vi "user process.vi"(8 "error in":errorcluster, 10 "Parameters to process":T2, 11 "Custom Temperature Controller runtime in":refnum<class "Custom Temperature Controller runtime.lvclass">) -> (0 "error out":errorcluster, 2 "Results from processing":T1, 3 "Custom Temperature Controller runtime out":refnum<class "Custom Temperature Controller runtime.lvclass">)   [LabVIEW 2021, in "Custom Temperature Controller runtime.lvclass"]
uses:
  Custom Temperature Controller runtime.lvclass
  parameter user data.ctl
  result user data.ctl
  Custom Temperature Controller runtime.lvclass/Custom Temperature Controller runtime.ctl
  <vilib>/addons/control/pid/pid.llb/PID (DBL).vi
  <vilib>/addons/control/pid/NI_PID_pid.lvlib
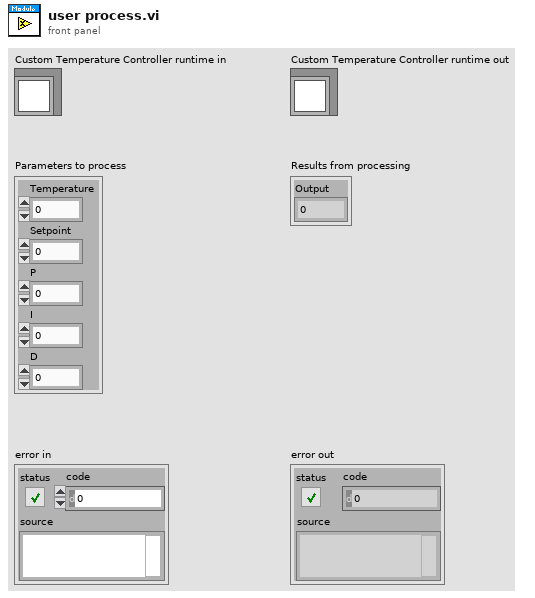
[diagram p1: front panel]
types:
  T1 = typedef "Custom Temperature Controller runtime.lvclass/result user data.ctl" = cluster{"Output":dbl}
  T2 = typedef "Custom Temperature Controller runtime.lvclass/parameter user data.ctl" = cluster{"Temperature":dbl, "Setpoint":dbl, "P":dbl, "I":dbl, "D":dbl}
  T3 = cluster{"proportional gain (Kc)":dbl, "integral time (Ti, min)":dbl, "derivative time (Td, min)":dbl}
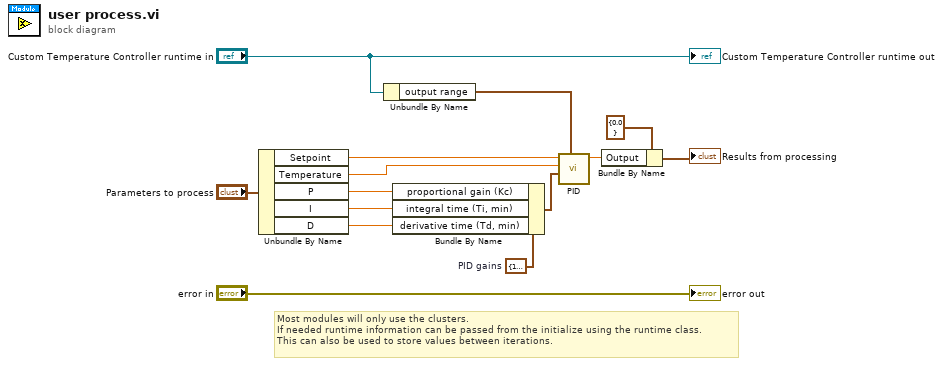
[diagram p0: block diagram]
diagram:
  w5 = T3 {"proportional gain (Kc)"=1.0, "integral time (Ti, min)"=0.01, "derivative time (Td, min)"=0.0}  # PID gains
  # "Most modules will only use the clusters.\nIf needed runtime information can be passed from the initialize using the runtime class.\nThis can also be used to store values between iterations."
  n1 = Unbundle By Name("Parameters to process") -> ("Setpoint"=w7:dbl, "Temperature"=w6:dbl, "P"=w3:dbl, "I"=w2:dbl, "D"=w1:dbl)
  n2 = Unbundle By Name("Custom Temperature Controller runtime in") -> ("output range"=w9:cluster{"output high":dbl, "output low":dbl})
  n3 = Bundle By Name(cluster=w5, "proportional gain (Kc)"=w3, "integral time (Ti, min)"=w2, "derivative time (Td, min)"=w1) -> (w4:T3)
  n4 = call-poly <vilib>:"PID.vi"("output range"=w9, "PID gains"=w4, "process variable"=w6, "setpoint"=w7) -> ("output"=w8:dbl)  [unwired: 6 in, 1 out]
  n5 = Bundle By Name(cluster=T1 {"Output"=0.0} ("Results from processing"), "Output"=w8) -> (→"Results from processing":T1)
  "error out" <- "error in"
  "Custom Temperature Controller runtime out" <- "Custom Temperature Controller runtime in"
